vi "PCO_RecorderInit.vi"(5 "szFilePath":path, 6 "wRamSegmentArr":u16[](array[numeric]), 7 "noOverwrite":bool, 8 "error in (no error)":errorcluster {"code" format="%x"}, 9 "wType":u16=1 min=1 max=4 step=1, 10 "dwImgCountArr":u32[](array[numeric]), 11 "phRec":u64) -> (0 "error out":errorcluster {"code" format="%x"}, 2 "ErrorMessage":i32 format="%x", 3 "phRec out":u64)   [LabVIEW 2019, in "Recorder.lvlib"]
doc: "<b>Description:</b>\nThis function initializes the recorder according to the required number of images for each camera. It will discard previous initializations.\n\nFor record-to-memory, it will allocate the RAM necessary to store the images. For record-to-file, it checks whether files with the same name are already existent and, depending on the wNoOverwrite flag either deletes the old files or if the flag is set, renames them. A file is renamed by adding (n) to the filename, where n is the lowest number that has not been contracted yet. This means, the higher the numbers in the brackets, the newer the files, but the file without brackets is always the newest/current one.\nThe function will be rejected with an error if an acquisition is running.\n\n<b>Supported camera type:</b>\nAll cameras"
uses:
  Recorder.lvlib
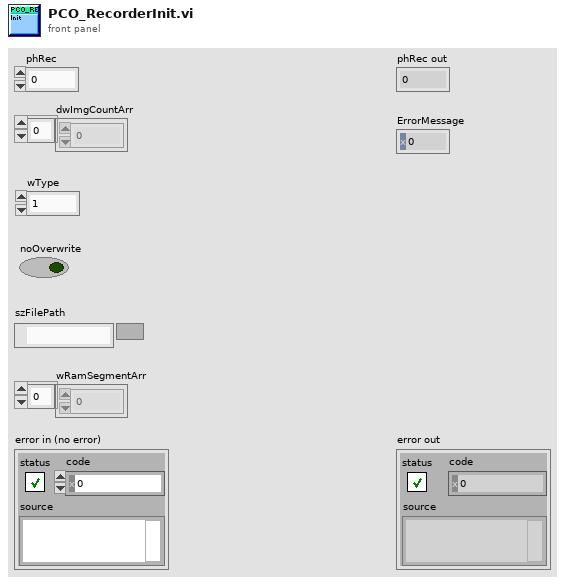
[diagram p1: front panel]
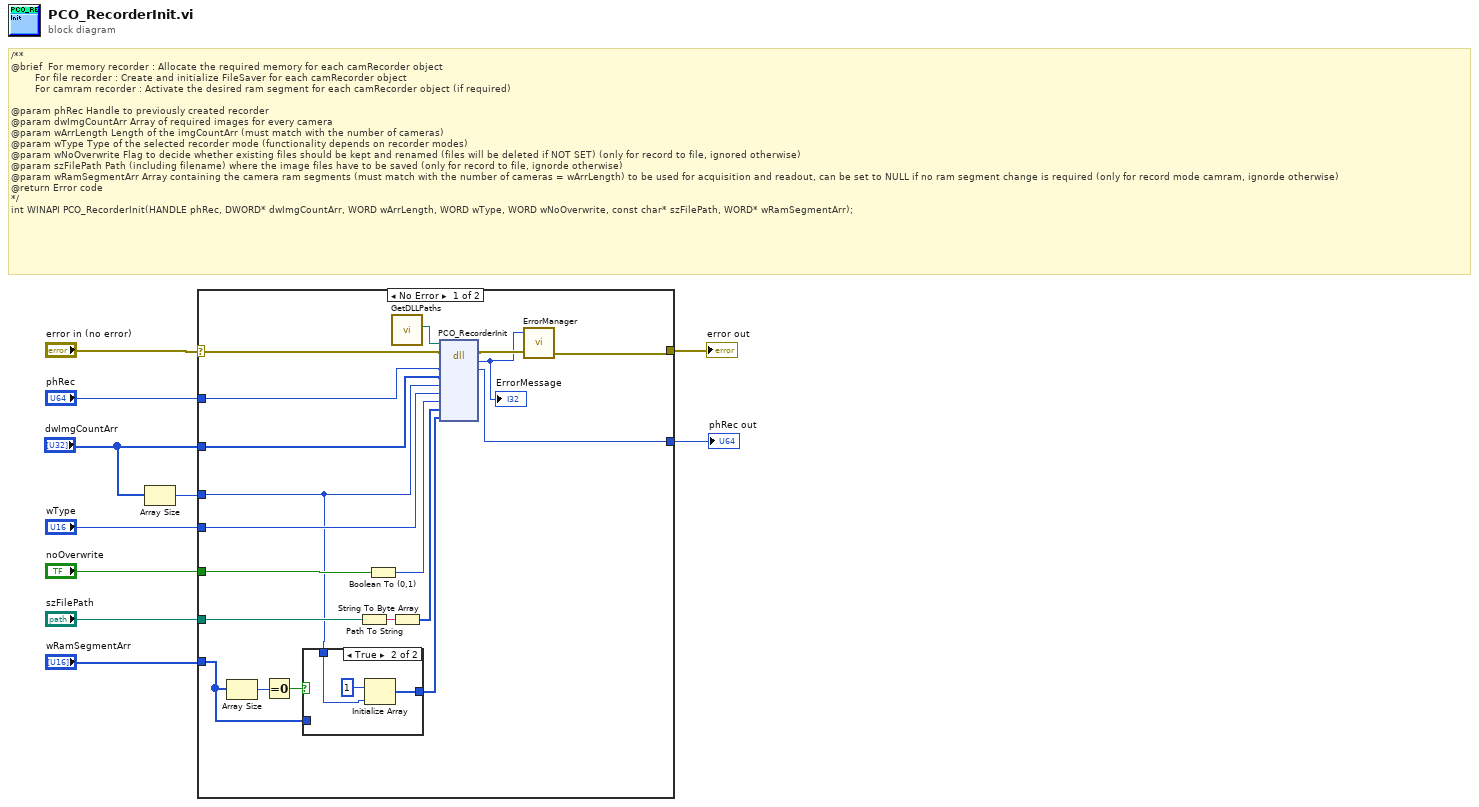
[diagram p0: block diagram]
diagram:
  # "/**\n@brief \tFor memory recorder : Allocate the required memory for each camRecorder object\n        For file recorder : Create and initialize FileSaver for each camRecorder object\n        For camram recorder : Activate the desired ram segment for each camRecorder object (if required)\n\n@param phRec Handle to previously created recorder\n@param dwImgCountArr Array of required images for every camera\n@param wArrLength Length of the imgCountArr (must match with the number of cameras)\n@param wType Type of the selected recorder mode (functionality depends on recorder modes)\n@param wNoOverwrite Flag to decide whether existing files should be kept and renamed (files will be deleted if NOT SET) (only for record to file, ignored otherwise)\n@param szFilePath Path (including filename) where the image files have to be saved (only for record to file, ignorde otherwise)\n@param wRamSegmentArr Array containing the camera ram segments (must match with the number of cameras = wArrLength) to be used for acquisition and readout, can be set to NULL if no ram segment change is required (only for record mode camram, ignorde otherwise)\n@return Error code\n*/\nint WINAPI PCO_RecorderInit(HANDLE phRec, DWORD* dwImgCountArr, WORD wArrLength, WORD wType, WORD wNoOverwrite, const char* szFilePath, WORD* wRamSegmentArr);"
  n1 = Array Size(array="dwImgCountArr") -> (size(s)=w3:i32)
  n2 = case shown="No Error" "error in (no error)" {
    selector: "error in (no error)" -> [w26 w35]
    tunnel: "phRec" -> [w24 w34]
    tunnel: [w25 w34] -> w9
    tunnel: "dwImgCountArr" -> [w23 _]
    tunnel: w3 -> [w11 _]
    tunnel: "noOverwrite" -> [w28 _]
    tunnel: "wType" -> [w22 _]
    tunnel: [w27 w35] -> w6
    tunnel: "szFilePath" -> [w29 _]
    tunnel: "wRamSegmentArr" -> [w13 _]
    frame No Error {
      n3 = Array Size(array=w13) -> (size(s)=w15:i32)
      n4 = Equal To 0?(x=w15) -> (x = 0?=w14:bool)
      n5 = case shown="True" w14 {
        tunnel: w13 -> [w30 _]
        tunnel: [w30 w32] -> w12
        tunnel: w11 -> [_ w31]
        frame False {
        }
        frame True {
          n6 = Initialize Array(u32 1 ("element"), w31) -> (w32:u32[])
        }
      }
      n7 = Path To String(path=w29) -> (string=w21:string)
      n8 = Boolean To (0,1)(Boolean=w28) -> (0, 1=w18:i16)
      n9 = call "GetDLLPaths.vi"() -> ("PCO_Recorder_Path"=w16:path)  [unwired: 9 in, 2 out]
      n10 = String To Byte Array(string=w21) -> (unsigned byte array=w17:u8[])
      n11 = dll-call lib="?" fn="PCO_RecorderInit"(path in=w16, error in=w26, "phRec"=w24, "dwImgCountArr"=w23, "wArrLength"=w11, "wType"=w22, "wNoOverwrite"=w18, "szFilePath"=w17, "wRamSegmentArr"=w12) -> (error out=w20:errorcluster, "return type"=w19:i32, "phRec"=w25:u64)  [unwired: 7 in, 1 out]
      "ErrorMessage" <- w19
      n12 = call "ErrorManager.vi"("error in (no error)"=w20, "error code"=w19) -> ("error out"=w27:errorcluster)  [unwired: 3 in]
    }
    frame Error {
    }
  }
  "phRec out" <- w9
  "error out" <- w6
